vi "ROS_Master_setMasterPort.vi"(2 "Port":u32=11311, 3 "Wait for real address?":bool, 4 "ROS_Master in":T1) -> (1 "ROS_Master out":T1)   [LabVIEW 2012]
doc: "Sets master port and checks for a valid connection"
uses:
  <userlib>/ROS for LabVIEW Software/ROS/Code/ROS_Master/ROS_Master.ctl
  <userlib>/ROS for LabVIEW Software/ROS/Code/ROS_Master/ROS_Topic.ctl
  <userlib>/ROS for LabVIEW Software/ROS/Code/ROS_Master/ROS_Node.ctl
  <userlib>/ROS for LabVIEW Software/ROS/Code/ROS_Master/ROS_Service.ctl
panel:
  out "Good?":bool
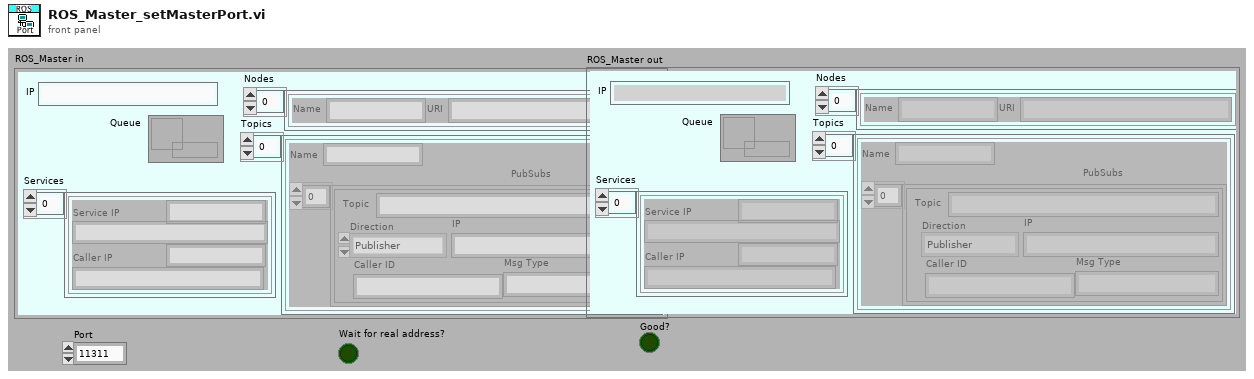
[diagram p1: front panel]
types:
  T1 = typedef "ROS_Master.ctl" = cluster{"IP":string, "Topics":cluster{"Name":string, "PubSubs":T2[]}[], "Nodes":T3[], "Services":T4[], "Queue":refnum<queue>}
  T2 = typedef "ROS_Topic.ctl" = cluster{"Caller ID":string, "IP":string, "Msg Type":string, "Direction":enum16{"Publisher", "Subscriber"}, "Topic":string}
  T3 = typedef "ROS_Node.ctl" = cluster{"Name":string, "URI":string}
  T4 = typedef "ROS_Service.ctl" = cluster{"Service":string, "Service IP":string, "Caller IP":string, "Caller ID":string}
  T5 = enum16{"http://IP:port", "http://IP", "IP:port", "IP only"}
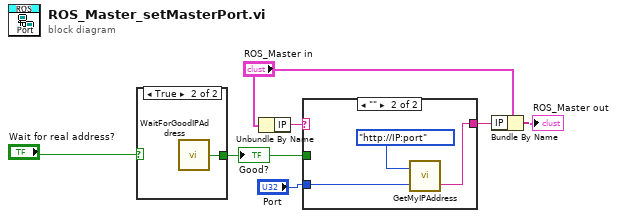
[diagram p0: block diagram]
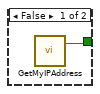
[diagram p2: hidden frame]
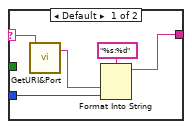
[diagram p3: hidden frame]
diagram:
  n1 = case shown="True" "Wait for real address?" {
    tunnel: [w8 w9] -> w1
    frame False {
      n2 = call <userlib>:"GetMyIPAddress.vi"() -> ("Good?"=w8:bool)  [unwired: 2 in, 1 out]
    }
    frame True {
      n3 = call <userlib>:"WaitForGoodIPAddress.vi"() -> ("Good?"=w9:bool)  [unwired: 1 in]
    }
  }
  "Good?" <- w1
  n4 = Unbundle By Name("ROS_Master in") -> ("IP"=w7:string)
  n5 = case shown="\"\"" w7 {
    selector: w7 -> [w11 _]
    tunnel: [w12 w16] -> w6
    tunnel: "Port" -> [w13 w17]
    tunnel: w1 -> [_ _]
    frame Default {
      n6 = call <userlib>:"GetURI&Port.vi"("URI in"=w11) -> ("URI"=w10:string)  [unwired: 1 out]
      n7 = Format Into String(format string="%s:%d", w10, w13) -> (resulting string=w12:string)  [unwired: 2 in, 1 out]
    }
    frame "" {
      n8 = call <userlib>:"GetMyIPAddress.vi"("Port"=w17, "Format"=T5."http://IP:port") -> ("URI"=w16:string)  [unwired: 1 out]
    }
  }
  n9 = Bundle By Name(cluster="ROS_Master in", "IP"=w6) -> (→"ROS_Master out":T1)
